vi "Image Transmitter.vi"() -> ()   [LabVIEW 2013]
uses:
  <vilib>/addons/Modulation/Digital/General/MT Generate PSK System Parameters(M).vi
  <vilib>/picture/picture.llb/Draw True-Color Pixmap.vi
  <instrlib>/niUSRP/niUSRP Write Tx Data (CDB Cluster).vi
  <vilib>/addons/Modulation/niDMT.lvlib
panel:
  in  "Scaling Factor":dbl(slide)=5.0 scale=0.0..10.0
  in  "Image File Path":path=path "E:/07/SUSTech-EE206-Communication-Principles-Laboratory/0528/Project_2/5/smiley_tiny(double).jpg"
  out "Transmitted Image":picture
  in  "Packet Parameters":T1={"Guard Bits "=30, "Sync Bits"=30, "Message Bits"=512}
  out "Number of Packets":i16=25000
  in  "Pulse Shaping Filter Parameters":T2={"Alpha"=0.5, "Filter Length"=6, "TX Filter"=enum."Root Raised Cos"} {"Alpha" format="%.2f"}
  out "Actual Tx Parameters":T3={"Tx IQ Sampling\nRate [s/sec]"=400000.0, "Tx Frequency [Hz]"=915000000.0, "Tx Gain [dB]"=20.0, "Tx Antenna"=""} {"Tx Gain [dB]" format="%#.6p"; "Tx Frequency [Hz]" format="%#.6p"; "Tx IQ Sampling\nRate [s/sec]" format="%#.6p"}
  in  "Tx Parameters":T3={"Tx IQ Sampling\nRate [s/sec]"=400000.0, "Tx Frequency [Hz]"=2330000000.0, "Tx Gain [dB]"=0.0, "Tx Antenna"="TX1"} {"Tx Gain [dB]" format="%#.6p"; "Tx Frequency [Hz]" format="%#.6p"; "Tx IQ Sampling\nRate [s/sec]" format="%#.6p"}
  in  "USRP IP Address":refnum<k15>="192.168.10.2"
  in  "Modulation Type":string(combo)="QPSK"
  out "Constellation Graph":T4(graph)
  out "Transmitted Signal":cluster{"t0":dbl, "dt":dbl, "Y":dbl[]}(graph)
  out "Error Out":errorcluster={"status"=FALSE, "code"=1074118647, "source"="niUSRP Fetch Rx Data (CDB Cluster).vi<ERR>Overflow: an internal receive buffer has filled before the data could be returned.  Consider reducing the IQ rate, increasing the Fetch rate, or increasing the number of samples per Fetch."}
  out "Symbol Rate [symbols/sec]":dbl=25000.0 format="%#.6p"
  in  "PN Sequence Order for Sync":i32=31
  in  "Stop":bool
  in  "Queue Length":i32=10
  in  "Packet Pad [samples]":i32=200
  in  "Blank Frame [samples]":i32=500
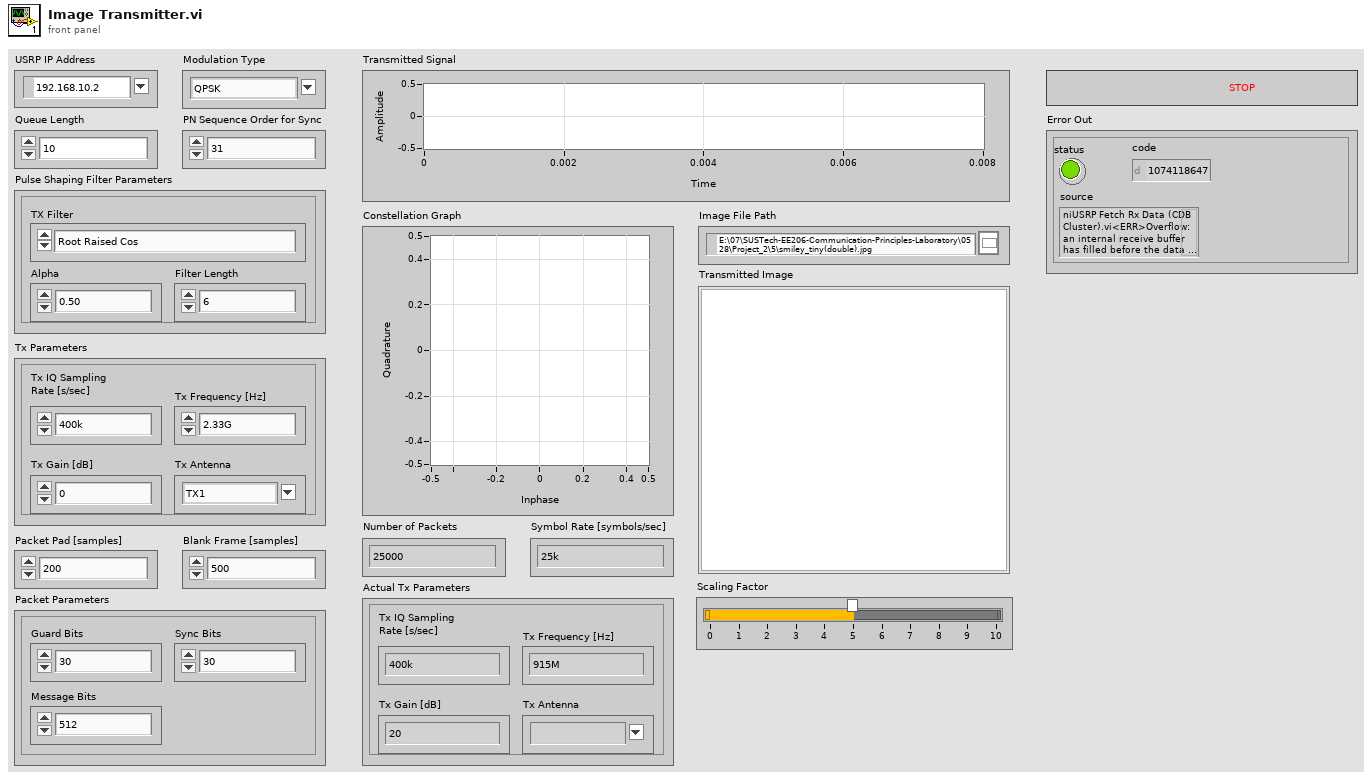
[diagram p1: front panel]
types:
  T1 = cluster{"Guard Bits ":i32, "Sync Bits":i32, "Message Bits":i32}
  T2 = cluster{"Alpha":dbl, "Filter Length":i32, "TX Filter":enum16{"none", "Raised Cosine", "Root Raised Cos", "Gaussian"}}
  T3 = cluster{"Tx IQ Sampling\nRate [s/sec]":dbl, "Tx Frequency [Hz]":dbl, "Tx Gain [dB]":dbl, "Tx Antenna":string}
  T4 = cluster{"constellation":dbl[], "oversampled data":dbl[]}[]
  T5 = typedef "imagedata.ctl" = cluster{"image type":i32, "image depth":i32, "image":u8[], "mask":u8[], "colors":u32[], "Rectangle":cluster{"left":i16, "top":i16, "right":i16, "bottom":i16}}
  T6 = cluster{"PSK type":u16, "Samples per Symbol":i32, "Differential PSK":enum16{"disable", "enable"}, "M":i32}
  T7 = cluster{"samples per symbol (16)":i32, "symbol map":cdb[], "differential PSK":enum16{"disable", "enable"}, "PSK type":u16}
  T8 = cluster{"s? t:f":cluster{"t0":dbl, "dt":dbl, "Y":cdb[]}, i32}
  T9 = cluster{"output complex waveform":cluster{"t0":dbl, "dt":dbl, "Y":cdb[]}, i32}
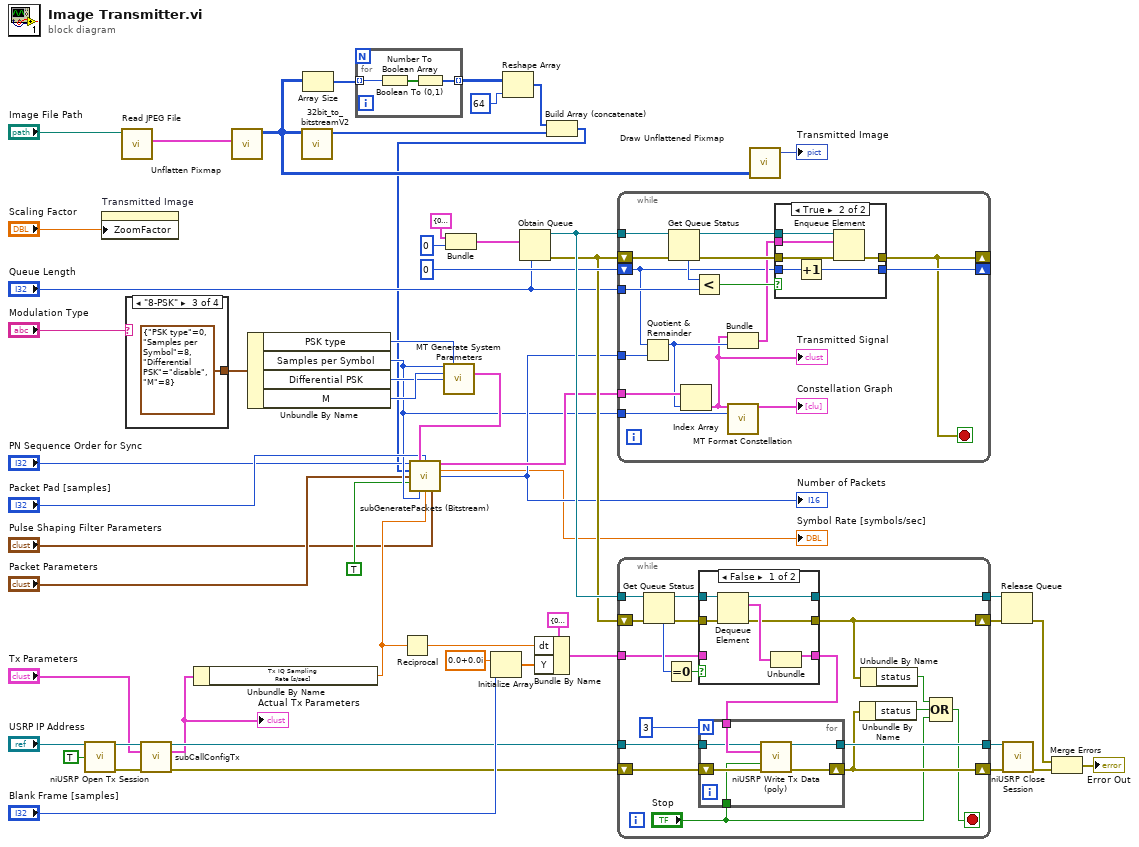
[diagram p0: block diagram]
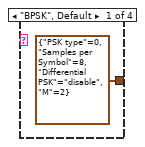
[diagram p2: hidden frame]
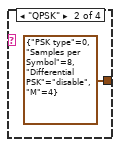
[diagram p3: hidden frame]
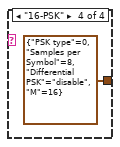
[diagram p4: hidden frame]
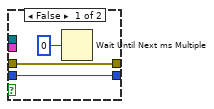
[diagram p5: hidden frame]
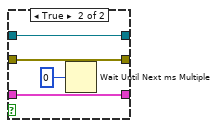
[diagram p6: hidden frame]
diagram:
  n1 = call <instrlib>:"niUSRP Open Tx Session.vi"("device names"="USRP IP Address", "reset"=TRUE) -> ("session handle out"=w37:refnum<k15>, "error out"=w36:errorcluster)  [unwired: 12 in]
  n2 = property on="Transmitted Image" class="Pict"("ZoomFactor"="Scaling Factor") -> ()  [unwired: 2 in, 2 out]
  n3 = call <vilib>:"Read JPEG File.vi"("path to JPEG file"="Image File Path") -> ("image data"=w21:T5)  [unwired: 8 in, 2 out]
  n4 = case shown="\"8-PSK\"" "Modulation Type" {
    tunnel: [T6 {"PSK type"=0, "Samples per Symbol"=8, "Differential PSK"=enum."disable", "M"=2} ("PSK Parameters") T6 {"PSK type"=0, "Samples per Symbol"=8, "Differential PSK"=enum."disable", "M"=4} ("PSK Parameters") T6 {"PSK type"=0, "Samples per Symbol"=8, "Differential PSK"=enum."disable", "M"=8} ("PSK Parameters") T6 {"PSK type"=0, "Samples per Symbol"=8, "Differential PSK"=enum."disable", "M"=16} ("PSK Parameters")] -> w27
    frame "BPSK", Default {
    }
    frame "QPSK" {
    }
    frame "8-PSK" {
    }
    frame "16-PSK" {
    }
  }
  n5 = call "subCallConfigTx.vi"("session handle"=w37, "Tx Parameters"="Tx Parameters", "error in"=w36) -> ("session handle out"=w41:refnum<k15>, "Actual Tx Parameters"=w32:T3, "error out"=w45:errorcluster)  [unwired: 10 in]
  "Actual Tx Parameters" <- w32
  n6 = Unbundle By Name(w32) -> ("Tx IQ Sampling\nRate [s/sec]"=w13:dbl)
  n7 = call <vilib>:"Unflatten Pixmap.vi"("image data"=w21) -> ("24-bit pixmap"=w7:u32[][])  [unwired: 4 in, 6 out]
  n8 = Unbundle By Name(w27) -> ("PSK type"=w26:u16, "Samples per Symbol"=w14:i32, "Differential PSK"=w24:enum16{"disable", "enable"}, "M"=w25:i32)
  n9 = call "32bit_to_bitstreamV2.vi"("24-bit pixmap"=w7) -> ("Bitstream with Guard"=w3:u8[])  [unwired: 7 in, 1 out]
  n10 = Array Size(array=w7) -> (size(s)=w6:i32[])
  n11 = for {
    tunnel: w6 -> [w62] mode=indexing
    tunnel: [w61] -> w4 mode=indexing
    n12 = Number To Boolean Array(number=w62) -> (Boolean array=w60:bool[])
    n13 = Boolean To (0,1)(Boolean=w60) -> (0, 1=w61:i16[])
  }
  n14 = Reciprocal(x=w13) -> (1/x=w42:dbl)
  n15 = call-poly <vilib>:"MT Generate System Parameters.vi"("samples per symbol (16)"=w14, "PSK type"=w26, "M-PSK (4)"=w25, "differential PSK"=w24) -> ("PSK system parameters"=w17:T7)  [unwired: 9 in, 2 out]
  n16 = Bundle("s? t:f"=cluster{"t0":dbl, "dt":dbl, "Y":cdb[]} {"t0"=0.0, "dt"=0.0, "Y"=[]}, 0) -> (w47:T8)  [unwired: 1 in]
  n17 = Initialize Array(cdb 0.0+0.0i ("element"), "Blank Frame [samples]") -> (w52:cdb[])
  n18 = Reshape Array(w4, 64) -> (w1:i16[])
  n19 = Obtain Queue(max queue size (-1, unlimited)="Queue Length", element data type=w47) -> (queue out=w53:refnum<queue>, error out=w39:errorcluster)  [unwired: 3 in, 1 out]
  n20 = Bundle By Name(cluster=cluster{"t0":dbl, "dt":dbl, "Y":cdb[]} {"t0"=0.0, "dt"=0.0, "Y"=[]} ("s? t:f"), "dt"=w42, "Y"=w52) -> (w51:cluster{"t0":dbl, "dt":dbl, "Y":cdb[]})
  n21 = Build Array (concatenate)(w1, w3) -> (w2:i16[])
  n22 = call "subGeneratePackets (Bitstream).vi"("PN sequence order\nfor Sync Bits"="PN Sequence Order for Sync", "PSK system parameters"=w17, "Packet Pad \n[samples]"="Packet Pad [samples]", "message bitstream"=w2, "Packet Parameters"="Packet Parameters", "Message Type"=TRUE, "Samples per Symbol"=w14, "Tx IQ Sampling\nRate [s/sec]"=w13, "Pulse Shaping Filter Parameters"="Pulse Shaping Filter Parameters") -> ("Packets"=w18:cluster{"t0":dbl, "dt":dbl, "Y":cdb[]}[], "Symbol Rate"=→"Symbol Rate [symbols/sec]":dbl, "Number of Packets"=w16:i32)  [unwired: 4 in]
  "Number of Packets" <- w16
  n23 = while {
    tunnel: w53 -> [w79]
    shift-right: [w72] -> _
    shift-left: 0 -> [w68]
    tunnel: w18 -> [w69]
    tunnel: "Queue Length" -> [w71]
    tunnel: w16 -> [w70]
    shift-right: [w66] -> _
    shift-left: w39 -> [w74]
    tunnel: w14 -> [w65]
    stop <- w66 stop-if-true
    n24 = Quotient & Remainder(x=w68, y=w70) -> (x-y*floor(x/y)=w67:i32)  [unwired: 1 out]
    n25 = Get Queue Status(queue=w79, error in (no error)=w74) -> (queue out=w78:refnum<queue>, error out=w75:errorcluster, # elements in queue=w77:i32)  [unwired: 1 in, 5 out]
    n26 = Index Array(array=w69, index=w67) -> (element=w63:cluster{"t0":dbl, "dt":dbl, "Y":cdb[]})
    "Transmitted Signal" <- w63
    n27 = Less?(x=w77, y=w71) -> (x < y?=w76:bool)
    n28 = Bundle("output complex waveform"=w63, w67) -> (w73:T9)  [unwired: 1 in]
    n29 = call <vilib>:"MT Format Constellation.vi"("waveform"=w63, "samples per symbol"=w65) -> ("constellation graph"=→"Constellation Graph":T4)  [unwired: 3 in, 10 out]
    n30 = case shown="True" w76 {
      tunnel: w75 -> [w80 w88]
      tunnel: w78 -> [_ w87]
      tunnel: [w80 w86] -> w66
      tunnel: w73 -> [_ w85]
      tunnel: w68 -> [w82 w84]
      tunnel: [w82 w83] -> w72
      frame False {
        n31 = Wait Until Next ms Multiple(millisecond multiple=u32 0) -> ()  [unwired: 1 out]
      }
      frame True {
        n32 = Increment(x=w84) -> (x+1=w83:i32)
        n33 = Enqueue Element(queue=w87, element=w85, error in (no error)=w88) -> (error out=w86:errorcluster)  [unwired: 1 in, 2 out]
      }
    }
  }
  n34 = while {
    tunnel: w41 -> [w98]
    shift-right: [w95] -> w44
    shift-left: w45 -> [w99]
    tunnel: w53 -> [w107]
    tunnel: w51 -> [w104]
    tunnel: [w103] -> w50
    tunnel: [w97] -> w43
    shift-right: [w92] -> w49
    shift-left: w39 -> [w100]
    stop <- w94 stop-if-true
    n35 = Get Queue Status(queue=w107, error in (no error)=w100) -> (queue out=w102:refnum<queue>, error out=w101:errorcluster, # elements in queue=w106:i32)  [unwired: 1 in, 5 out]
    n36 = Equal To 0?(x=w106) -> (x = 0?=w105:bool)
    n37 = case shown="False" w105 {
      tunnel: w104 -> [_ w123]
      tunnel: [w115 w123] -> w90
      tunnel: [w119 w121] -> w103
      tunnel: [w114 w122] -> w92
      tunnel: w102 -> [w118 w121]
      tunnel: w101 -> [w117 w122]
      frame False {
        n38 = Dequeue Element(queue=w118, error in (no error)=w117) -> (queue out=w119:refnum<queue>, element=w116:T8, error out=w114:errorcluster)  [unwired: 1 in, 1 out]
        n39 = Unbundle(w116) -> ("s? t:f"=w115:cluster{"t0":dbl, "dt":dbl, "Y":cdb[]})  [unwired: 1 out]
      }
      frame True {
        n40 = Wait Until Next ms Multiple(millisecond multiple=u32 0) -> ()  [unwired: 1 out]
      }
    }
    n41 = for {
      N: 3 -> [_]
      tunnel: w90 -> [w112]
      tunnel: w98 -> [w111]
      tunnel: [w110] -> w97
      tunnel: "Stop" -> [w109]
      shift-right: [w108] -> w95
      shift-left: w99 -> [w113]
      n42 = call-poly <instrlib>:"niUSRP Write Tx Data (poly).vi"("session handle"=w111, "data"=w112, "end of data?"=w109, "error in (no error)"=w113) -> ("session handle out"=w110:refnum<k15>, "error out"=w108:errorcluster)  [unwired: 10 in]
    }
    n43 = Unbundle By Name(w95) -> ("status"=w96:bool)
    n44 = Unbundle By Name(w92) -> ("status"=w91:bool)
    n45 = Compound Arithmetic op=OR(w91, w96, "Stop") -> (w94:bool)
  }
  n46 = call-poly <vilib>:"Draw Unflattened Pixmap.vi"("data (RGB format)"=w7) -> ("new picture"=→"Transmitted Image":picture)  [unwired: 8 in]
  n47 = Release Queue(queue=w50, error in (no error)=w49) -> (error out=w23:errorcluster)  [unwired: 3 out]
  n48 = call <instrlib>:"niUSRP Close Session.vi"("session handle"=w43, "error in (no error)"=w44) -> ("error out"=w35:errorcluster)  [unwired: 13 in]
  n49 = Merge Errors(w23, w35) -> (→"Error Out":errorcluster)
